vi "VINameEscape.vi"(11 "label":string) -> (3 "escaped string":string)   [LabVIEW 2019, in "SetGetControlValue.lvlib"]
uses:
  SetGetControlValue.lvlib
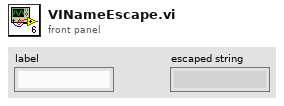
[diagram p1: front panel]
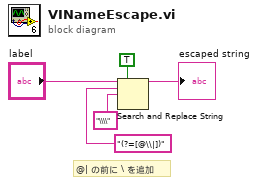
[diagram p0: block diagram]
diagram:
  # "@| の前に \\ を追加"
  n1 = Search and Replace String(replace all?=TRUE ("replace all? (F)"), input string="label", search string="(?=[@\\|])", replace string="\\\\" ("replace string (\"\")")) -> (result string=→"escaped string":string)  [unwired: 4 in, 3 out]
